vi "Unique Node Values.vi"(10 "Array B":string[](array[string]), 11 "Array A":string[](array[string])) -> (3 "Array out":string[](array[string]))   [LabVIEW 2025]
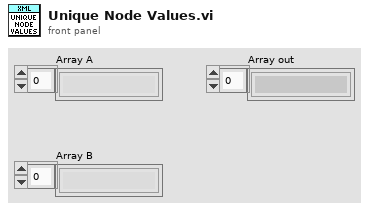
[diagram p1: front panel]
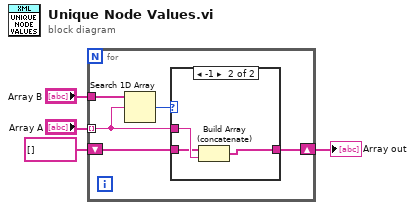
[diagram p0: block diagram]
diagram:
  n1 = for {
    tunnel: "Array A" -> [w7] mode=indexing
    tunnel: "Array B" -> [w9]
    shift-right: [w5] -> w1
    shift-left: string[] [] -> [w6]
    n2 = Search 1D Array(1D array=w9, element=w7) -> (index of element=w8:i32)  [unwired: 1 in]
    n3 = case shown="-1" w8 {
      tunnel: w7 -> [_ w13]
      tunnel: w6 -> [w10 w12]
      tunnel: [w10 w11] -> w5
      frame 0, Default {
      }
      frame -1 {
        n4 = Build Array (concatenate)(w12, w13) -> (w11:string[])
      }
    }
  }
  "Array out" <- w1
